vi "Sets_Unique(LVObject).vi"(8 "error in (no error)":errorcluster caption="错误输入（无错误）", 11 "输入数组":refnum<class>[](array[class])) -> (0 "error out":errorcluster caption="错误输出", 2 "已删除元素索引":i32[](array[numeric]), 3 "输出数组":refnum<class>[](array[class]))   [LabVIEW 2013]
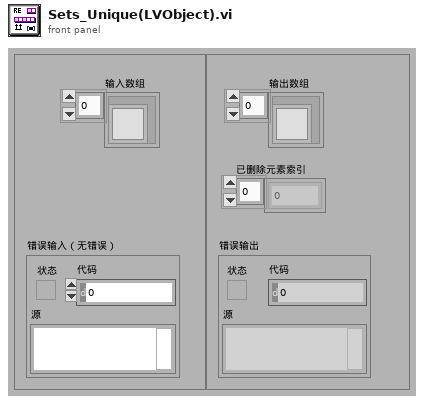
[diagram p1: front panel]
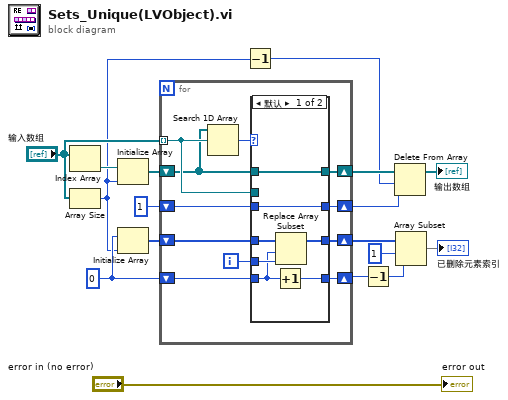
[diagram p0: block diagram]
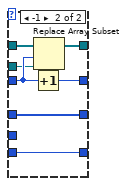
[diagram p2: hidden frame]
diagram:
  w11 = 0
  n1 = Index Array(array="输入数组") -> (element=w17:refnum<class>)  [unwired: 1 in]
  n2 = Array Size(array="输入数组") -> (size(s)=w8:i32)
  n3 = Initialize Array(w17, w8) -> (w15:refnum<class>[])
  n4 = Initialize Array(w11, w8) -> (w12:i32[])
  n5 = for {
    tunnel: "输入数组" -> [w25] mode=indexing
    shift-right: [w23] -> w10
    shift-left: w15 -> [w24]
    shift-right: [w26] -> w9
    shift-left: 1 -> [w27]
    shift-right: [w19] -> w7
    shift-left: w12 -> [w22]
    shift-right: [w20] -> w6
    shift-left: w11 -> [w21]
    i -> [w18]
    n6 = Search 1D Array(1D array=w24, element=w25) -> (index of element=w28:i32)  [unwired: 1 in]
    n7 = case shown="默认" w28 {
      tunnel: w27 -> [w35 w41]
      tunnel: [w35 w42] -> w26
      tunnel: w25 -> [_ w40]
      tunnel: w24 -> [w34 w39]
      tunnel: [w34 w38] -> w23
      tunnel: w22 -> [w32 w37]
      tunnel: w21 -> [w29 w36]
      tunnel: [w33 w36] -> w20
      tunnel: [w31 w37] -> w19
      tunnel: w18 -> [w30 _]
      frame Default {
        n8 = Increment(x=w29) -> (x+1=w33:i32)
        n9 = Replace Array Subset(array=w32, new element=w30, index=w29) -> (w31:i32[])
      }
      frame -1 {
        n10 = Increment(x=w41) -> (x+1=w42:i32)
        n11 = Replace Array Subset(array=w39, new element=w40, index=w41) -> (w38:refnum<class>[])
      }
    }
  }
  n12 = Decrement(x=w8) -> (x-1=w5:i32)
  n13 = Decrement(x=w6) -> (x-1=w1:i32)
  n14 = Delete From Array(array=w10, length=w5, index=w9) -> (array with subset deleted=→"输出数组":refnum<class>[])  [unwired: 1 out]
  n15 = Array Subset(array=w7, index=1 ("索引"), length=w1) -> (→"已删除元素索引":i32[])
  "error out" <- "error in (no error)"
